vi "4Pi Interference Locator.vi"() -> ()   [LabVIEW 2016]
uses:
  Hardware Configuration/Hardware Configuration Controls/Device Type.ctl
  Hardware Configuration/Hardware Configuration Controls/Device Function.ctl
  Device Library/Stages/Stages Controls/Stage Status.ctl
  Device Library/Stages/Stages Controls/Stage Actions.ctl
  <vilib>/vision/NI_Vision_Development_Module.lvlib
panel:
  out "error out 2":errorcluster
  out "error out":errorcluster
  out "Quad 01 Image":T1(plugin-control)
  in  "clear first (no:F)":bool
  out "Position":dbl
  in  "Abort":bool
  in  "Move":bool
  out "XY Graph":cluster{"X":dbl, "Y":dbl}[](graph)
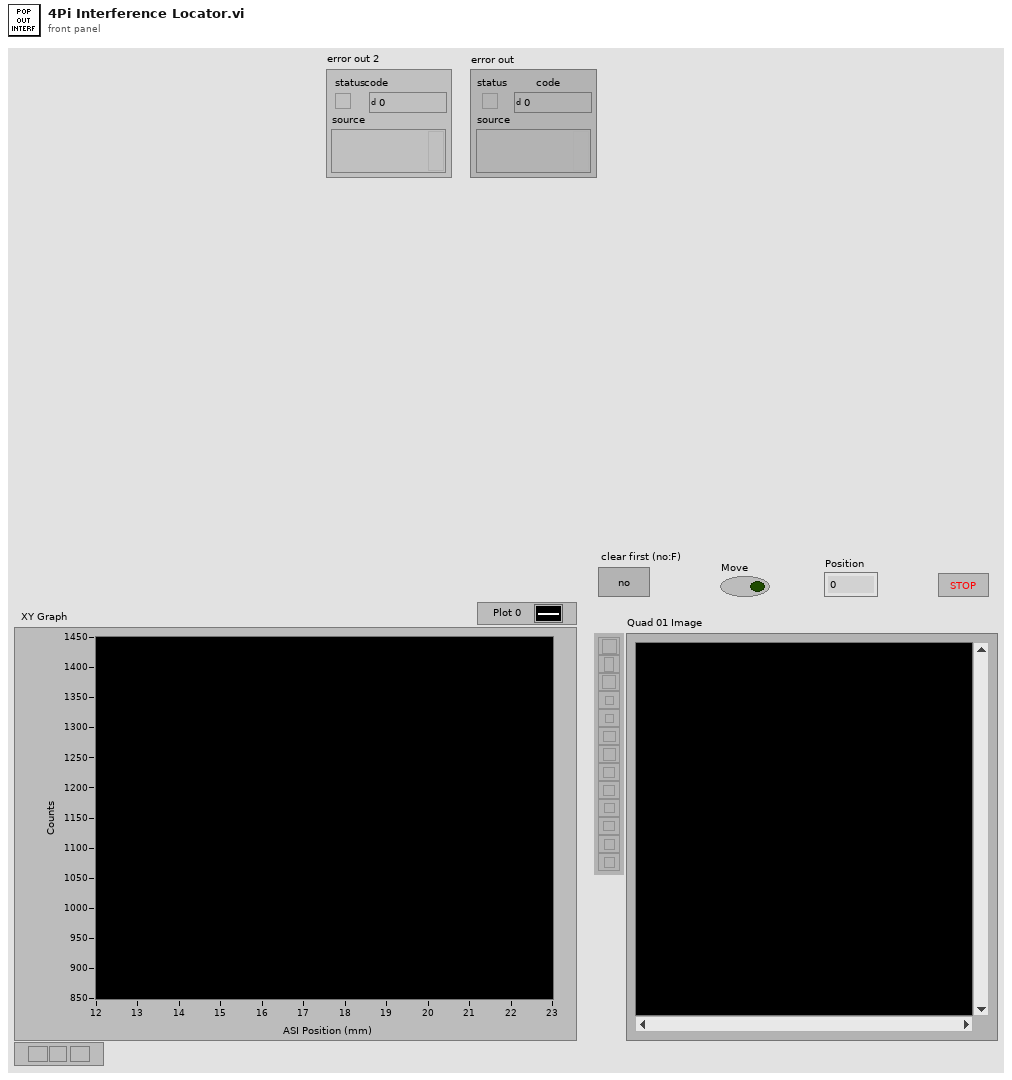
[diagram p1: front panel]
types:
  T1 = typedef "IMAQ Image.ctl" = refnum<image>
  T2 = typedef "Device Function.ctl" = enum16{"Primary", "Secondary", "Overview", "Wide Field Drift Correction", "642 nm Excitation", "560 nm Excitation", "546 nm Excitation", "488 nm Excitation", "405 nm Excitation", "Objective Drift Correction", "Objective XY", "Objective Z", "Sample XY", "Sample Coarse Z", "Sample Z", "4Pi Lower", "4Pi Upper", "Adj Cavity"}
  T3 = typedef "Device Type.ctl" = enum16{"AOTF", "Camera", "Deformable Mirror", "Laser", "Shutter", "Stage"}
  T4 = typedef "Image Type" = u32
  T5 = typedef "Stage Actions.ctl" = enum16{"Get Position", "MVR", "MOVE", "HALT", "ONTARGET", "ERROR", "REFERENCE", "INIT", "VELOCITY", "STATUS", "EXIT", "HOME", "ZEROPOS", "NANOPOS", "ANALOG", "QUIT"}
  T6 = typedef "Stage Status.ctl" = enum16{"Error", "Abort", "Busy", "On Target"}
  T7 = cluster{"Global Rectangle":i32[], "Contours":cluster{"Contour Type":u32, "ROI Type":u32, "Points":i32[]}[]}
  T8 = cluster{"Contour Type":u32, "ROI Type":u32, "Points":i32[]}[]
  T9 = cluster{"Contour Type":u32, "ROI Type":u32, "Points":i32[]}
  T10 = cluster{"Mean Value":sgl, "Standard Variation":sgl, "Minimal Value":sgl, "Maximal Value":sgl, "Area (calibrated)":sgl, "Area (pixels)":u32, "%":sgl, "Calibration Valid":bool}
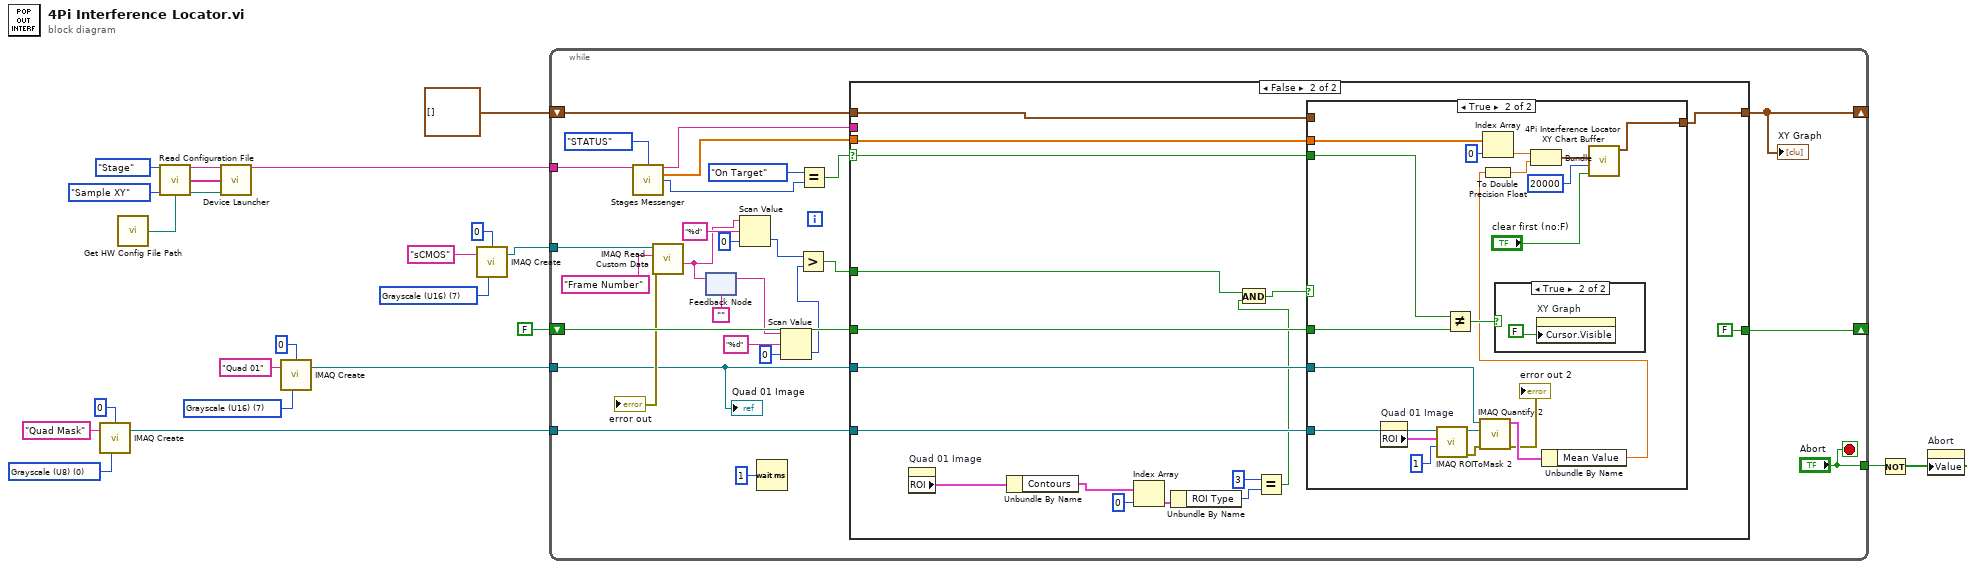
[diagram p0: block diagram]
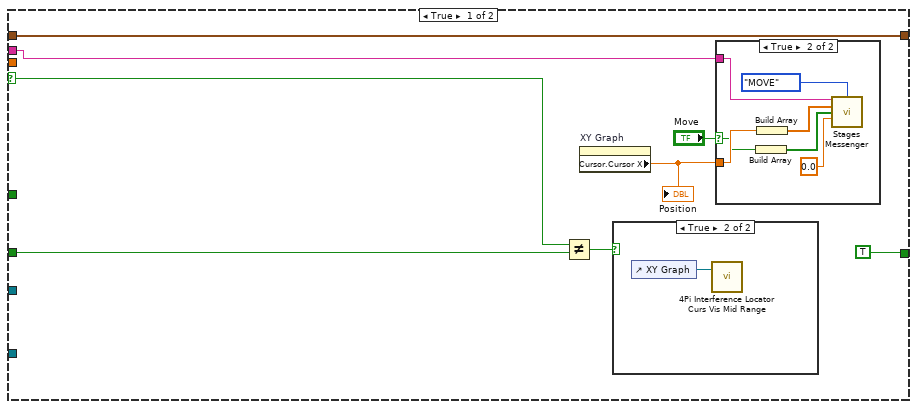
[diagram p2: hidden frame]
diagram:
  w11 = T4 7 items=["Grayscale (U8)", "Grayscale (I16)", "Grayscale (SGL)", "Complex (CSG)", "RGB (U32)", "HSL (U32)", "RGB (U64)", "Grayscale (U16)"] ("Image Type")
  w14 = T4 0 items=["Grayscale (U8)", "Grayscale (I16)", "Grayscale (SGL)", "Complex (CSG)", "RGB (U32)", "HSL (U32)", "RGB (U64)", "Grayscale (U16)"] ("Image Type")
  w18 = T4 7 items=["Grayscale (U8)", "Grayscale (I16)", "Grayscale (SGL)", "Complex (CSG)", "RGB (U32)", "HSL (U32)", "RGB (U64)", "Grayscale (U16)"] ("Image Type")
  n1 = call "IMAQ Create"("Border Size"=0, "Image Name"="Quad Mask", "Image Type"=w14) -> ("New Image"=w12:T1)  [unwired: 2 in, 1 out]
  n2 = call "Get HW Config File Path.vi"() -> ("File Path"=w2:path)  [unwired: 14 in, 1 out]
  n3 = call "Read Configuration File.vi"("Device Type"=Device_Type."Stage", "Device Function"=Device_Function."Sample XY", "Config File Path"=w2) -> ("Unique Notifier Name"=w7:string, "Device Ports/IDs/Channels"=w5:string[], "Device Engine Path"=w6:path)  [unwired: 9 in, 1 out]
  n4 = call "Device Launcher.vi"("Notifier Name"=w7, "Device Ports/IDs/Channels"=w5, "Device Engine Path"=w6) -> ("Notifier Name"=w1:string)  [unwired: 11 in, 1 out]
  n5 = call "IMAQ Create"("Border Size"=0, "Image Name"="Quad 01", "Image Type"=w18) -> ("New Image"=w16:T1)  [unwired: 2 in, 1 out]
  n6 = call "IMAQ Create"("Border Size"=0, "Image Name"="sCMOS" ("name (unnamed)"), "Image Type"=w11) -> ("New Image"=w8:T1)  [unwired: 2 in, 1 out]
  n7 = while {
    shift-right: [w51] -> _
    shift-left: cluster{"x":dbl, "y":dbl}[] [] ("XY chart data") -> [w50]
    tunnel: ["Abort"] -> w22
    shift-right: [w49] -> _
    shift-left: FALSE -> [w48]
    tunnel: w16 -> [w29]
    tunnel: w12 -> [w47]
    tunnel: w8 -> [w44]
    tunnel: w1 -> [w27]
    stop <- "Abort" stop-if-true
    n8 = call "Stages Messenger.vi"("Stage Notifier Name"=w27, "Actions"=Stage_Actions."STATUS") -> ("Stage Notifier Name (Dup)"=w24:string, "Positions"=w26:dbl[], "Status"=w25:T6)  [unwired: 10 in, 1 out]
    n9 = call "IMAQ Read Custom Data"("Key"="Frame Number", "Image"=w44) -> ("error out"=→"error out":errorcluster, "Custom Data Out"=w35:string)  [unwired: 7 in, 1 out]
    n10 = feedback-in #1(w35) -> ()
    n11 = feedback #1("") -> (w32:string)
    n12 = Scan Value(string=w35, format string="%d", default (0 dbl)=u32 0) -> (value=w31:u32)  [unwired: 1 out]
    n13 = Wait (ms)(milliseconds to wait=u32 1) -> ()  [unwired: 1 out]
    n14 = Scan Value(string=w32, format string="%d", default (0 dbl)=u32 0) -> (value=w30:u32)  [unwired: 1 out]
    n15 = Greater?(x=w31, y=w30) -> (0:w43:bool)
    n16 = Equal?(x=Stage_Status."On Target", y=w25) -> (x = y?=w40:bool)
    n17 = case shown="False" w40 {
      selector: w40 -> [w55 w80]
      tunnel: [w59 w84] -> w51
      tunnel: w50 -> [w59 w77]
      tunnel: w26 -> [_ w83]
      tunnel: [TRUE FALSE] -> w49
      tunnel: w48 -> [w54 w81]
      tunnel: w47 -> [_ w79]
      tunnel: w29 -> [_ w78]
      tunnel: w43 -> [_ w70]
      tunnel: w24 -> [w52 _]
      frame True {
        n18 = Not Equal?(x=w55, y=w54) -> (x != y?=w53:bool)
        n19 = property on="XY Graph" class="XYGraph (strict)"() -> ("Cursor.Cursor X"=w58:dbl)  [unwired: 2 in, 2 out]
        "Position" <- w58
        n20 = case shown="True" w53 {
          frame False {
          }
          frame True {
            n21 = control-ref of="XY Graph"() -> (w60:refnum<vi>)
            n22 = call "4Pi Interference Locator Curs Vis Mid Range.vi"("XYGraph in"=w60) -> ()  [unwired: 11 in]
          }
        }
        n23 = case shown="True" "Move" {
          selector: "Move" -> [_ w65]
          tunnel: w58 -> [_ w67]
          tunnel: w52 -> [_ w61]
          frame False {
          }
          frame True {
            n24 = Build Array(w65) -> (w64:bool[])
            n25 = Build Array(w67) -> (w66:dbl[])
            n26 = call "Stages Messenger.vi"("Stage Notifier Name"=w61, "Actions"=Stage_Actions."MOVE" ("Action"), "Setpoint"=w66, "Axis"=w64, "Velocity"=0.0) -> ()  [unwired: 7 in, 4 out]
          }
        }
      }
      frame False {
        n27 = property on="Quad 01 Image" class="ImageControl"() -> ("ROI"=w76:T7)  [unwired: 2 in, 2 out]
        n28 = Unbundle By Name(w76) -> ("Contours"=w75:T8)
        n29 = Index Array(array=w75, index=0) -> (element=w73:T9)
        n30 = Unbundle By Name(w73) -> ("ROI Type"=w72:u32)
        n31 = Equal?(x=u32 3, y=w72) -> (x = y?=w69:bool)
        n32 = And(x=w70, y=w69) -> (x .and. y?=w68:bool)
        n33 = case shown="True" w68 {
          tunnel: [w85 w103] -> w84
          tunnel: w83 -> [_ w100]
          tunnel: w81 -> [_ w98]
          tunnel: w80 -> [_ w97]
          tunnel: w79 -> [_ w92]
          tunnel: w78 -> [_ w88]
          tunnel: w77 -> [w85 _]
          frame False {
          }
          frame True {
            n34 = property on="Quad 01 Image" class="ImageControl"() -> ("ROI"=w91:T7)  [unwired: 2 in, 2 out]
            n35 = call "IMAQ ROIToMask 2"("Filling Value (255)"=1, "ROI Descriptor"=w91, "Image"=w92) -> ("error out"=w87:errorcluster, "Image Out"=w94:T1)  [unwired: 6 in, 1 out]
            n36 = Not Equal?(x=w97, y=w98) -> (x != y?=w96:bool)
            n37 = call "IMAQ Quantify 2"("error in (no error)"=w87, "Image Mask"=w94, "Image"=w88) -> ("error out"=→"error out 2":errorcluster, "Global Report"=w90:T10)  [unwired: 6 in, 1 out]
            n38 = Index Array(array=w100, index=0) -> (element=w99:dbl)
            n39 = case shown="True" w96 {
              frame False {
              }
              frame True {
                n40 = property on="XY Graph" class="XYGraph (strict)"("Cursor.Visible"=FALSE) -> ()  [unwired: 2 in, 2 out]
              }
            }
            n41 = Unbundle By Name(w90) -> ("Mean Value"=w89:sgl)
            n42 = To Double Precision Float(number=w89) -> (double precision float=w104:dbl)
            n43 = Bundle("Position"=w99, w104) -> (w105:cluster{"Position":dbl, dbl})  [unwired: 1 in]
            n44 = call "4Pi Interference Locator XY Chart Buffer.vi"("clear first (no:F)"="clear first (no:F)", "chart length (points)"=20000, "new point"=w105) -> ("XY chart data"=w103:cluster{"x":dbl, "y":dbl}[])  [unwired: 8 in]
          }
        }
      }
    }
    "XY Graph" <- w51
    "Quad 01 Image" <- w29
  }
  n45 = Not(x=w22) -> (.not. x?=w21:bool)
  n46 = property on="Abort" class="Bool (strict)"("Value"=w21) -> ()  [unwired: 2 in, 2 out]
